vi "624 Detect Retroreflective Vision Totes.vi"(7 "Limit %":dbl=0.5 format="%#_13g", 8 "Filter Settings":T2, 9 "Ring Light Color":T4={"Hue"={101.37467765958063, 64.10933859299683}, "Sat"={88.03571428571429, 255.0}, "Val"={133.57142857142858, 255.0}} {"Hue" scale=0.0..255.0 scale format="%#_3g"}, 10 "Image Src":T3, 11 "Camera FOV width":dbl) -> (1 "Detected totes":T1[](array[typedef]), 2 "Masked":T3(plugin-control), 3 "Processed Img":T3(plugin-control))   [LabVIEW 2014]
uses:
  <vilib>/vision/Image Controls.llb/IMAQ Image.ctl
  Particle Filter Settings.ctl
  Vision Tote Data.ctl
  <vilib>/vision/NI_Vision_Development_Module.lvlib
panel:
  in  "Aspect Fudge Factor":dbl=1.0
  out "ms to process":u32
  out "Particles":i32
  # "Instructions:\nUse Source to select image files from a directory or use a USB or IP camera connected to your laptop.\nUse the Color of a ring light to threshold and build particles. Adjust calibration if needed.\nSmall modifications to the diagram will allow for intensity processing instead of color.\nAnnotations show the rectangle and the scores from top to bottom."
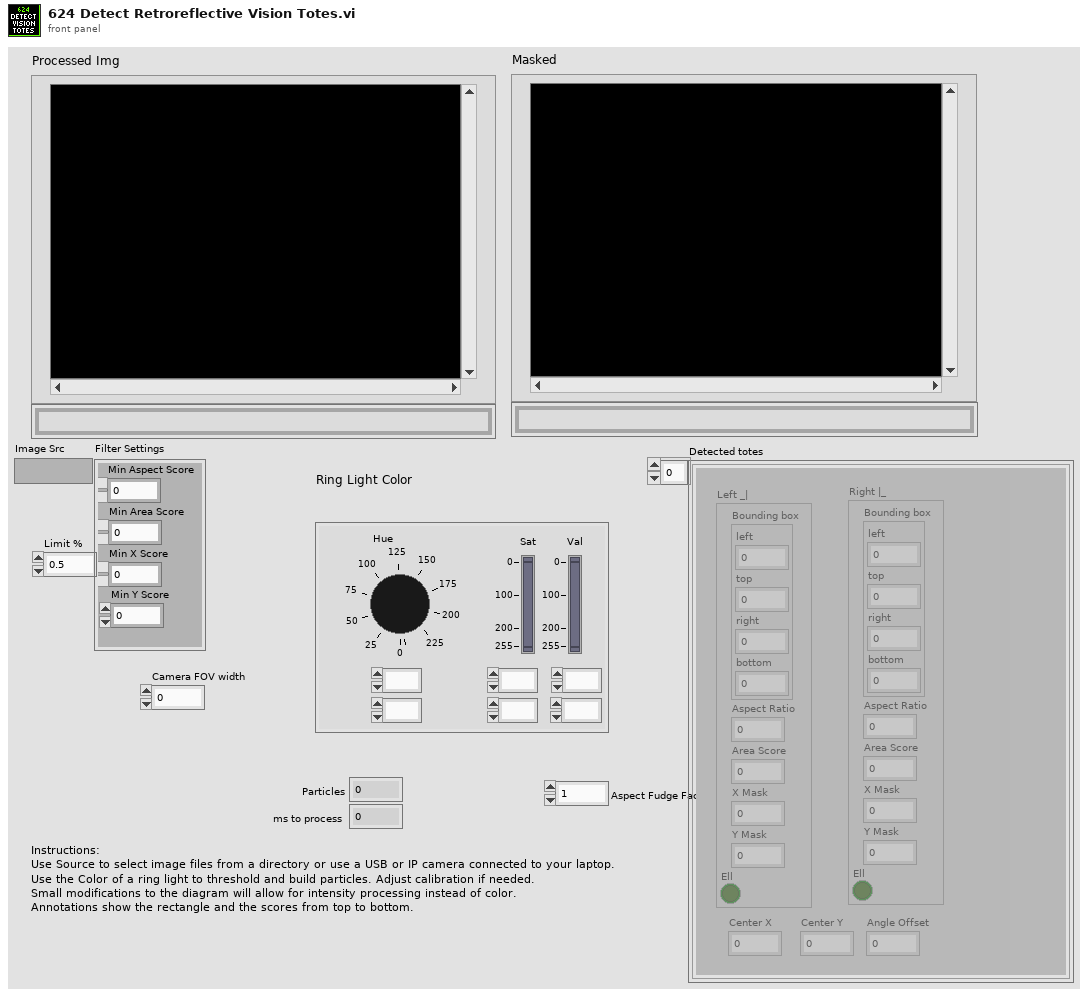
[diagram p1: front panel]
types:
  T1 = typedef "Vision Tote Data.ctl" = cluster{"Left _|":cluster{"Bounding box":cluster{"left":dbl, "top":dbl, "right":dbl, "bottom":dbl}, "Aspect Ratio":dbl, "Area Score":dbl, "X Mask":dbl, "Y Mask":dbl, "Ell":bool}, "Right |_":cluster{"Bounding box":cluster{"left":dbl, "top":dbl, "right":dbl, "bottom":dbl}, "Aspect Ratio":dbl, "Area Score":dbl, "X Mask":dbl, "Y Mask":dbl, "Ell":bool}, "Center X":dbl, "Center Y":dbl, "Angle Offset":dbl}
  T2 = typedef "Particle Filter Settings.ctl" = cluster{"Min Aspect Score":dbl, "Min Area Score":dbl, "Min X Score":dbl, "Min Y Score":dbl}
  T3 = typedef "IMAQ Image.ctl" = refnum<image>
  T4 = cluster{"Hue":cluster{dbl, dbl}, "Sat":cluster{dbl, dbl}, "Val":cluster{dbl, dbl}}
  T5 = typedef "Particle Parameters" = i32
  T6 = typedef "Image Type" = u32
  T7 = cluster{"Bounding box":cluster{"left":dbl, "top":dbl, "right":dbl, "bottom":dbl}, "Aspect Ratio":dbl, "Area Score":dbl, "X Mask":dbl, "Y Mask":dbl, "Ell":bool}[]
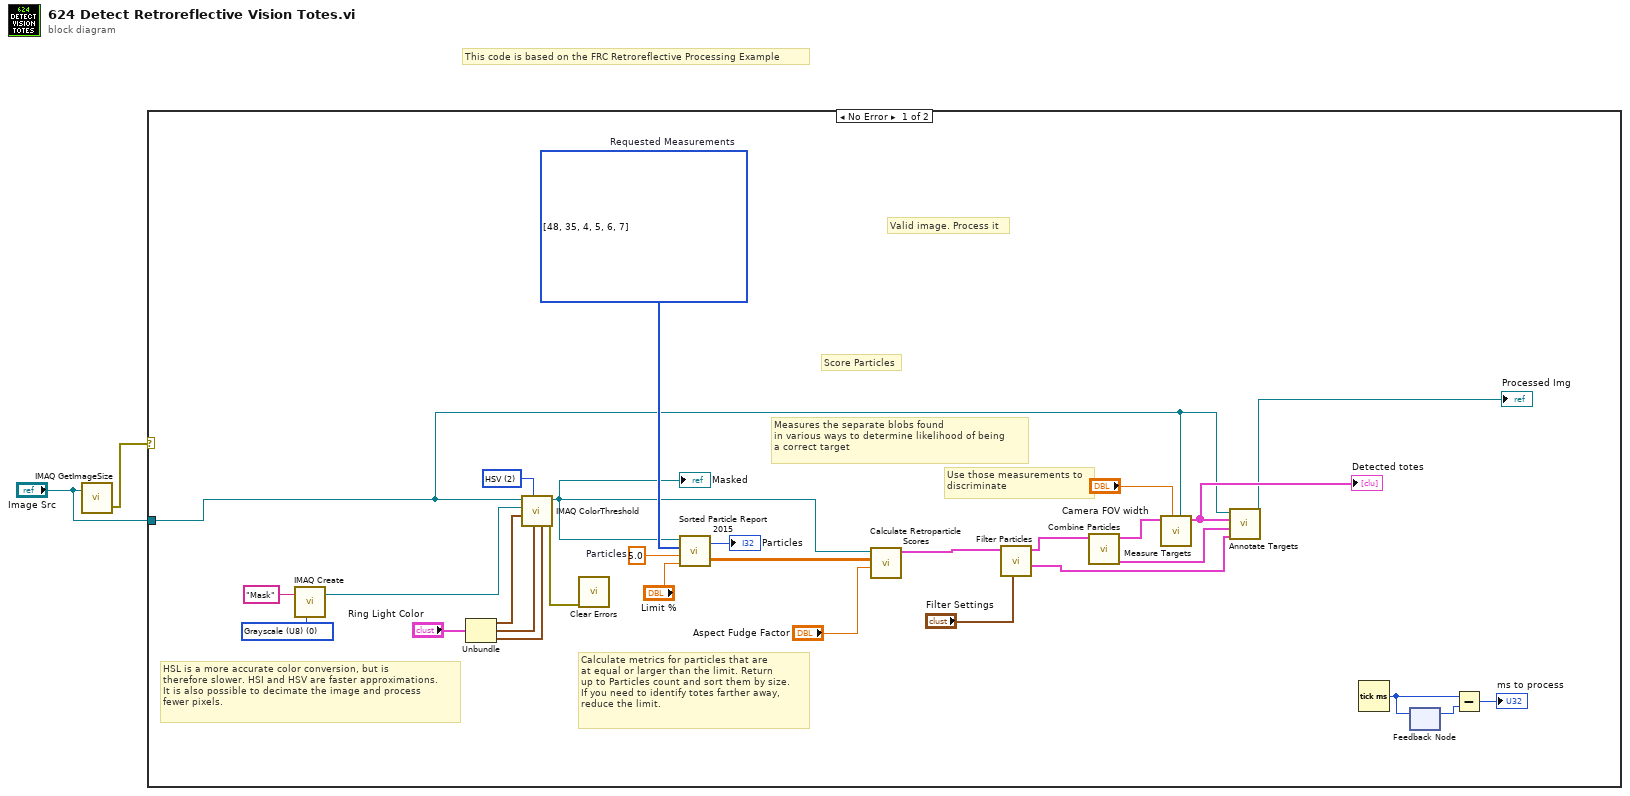
[diagram p0: block diagram]
diagram:
  # "This code is based on the FRC Retroreflective Processing Example"
  n1 = call "IMAQ GetImageSize"("Image"="Image Src") -> ("error out"=w1:errorcluster)  [unwired: 3 in, 2 out]
  n2 = case shown="No Error" w1 {
    tunnel: "Image Src" -> [w4 _]
    frame No Error {
      w22 = 5.0  # Particles
      w27 = u16 2 items=["RGB", "HSL", "HSV", "HSI"] ("Color Mode")
      w28 = T5[] [48, 35, 4, 5, 6, 7] items=["Center of Mass X", "Center of Mass Y", "First Pixel X", "First Pixel Y", "Bounding Rect Left", "Bounding Rect Top", "Bounding Rect Right", "Bounding Rect Bottom", "Max Feret Diameter Start X", "Max Feret Diameter Start Y", "Max Feret Diameter End X", "Max Feret Diameter End Y", "Max Horiz. Segment Length Left", "Max Horiz. Segment Length Right", "Max Horiz. Segment Length Row", "-", "Bounding Rect Width", "Bounding Rect Height", "Bounding Rect Diagonal", "Perimeter", "Convex Hull Perimeter", "Holes' Perimeter", "Max Feret Diameter", "Equivalent Ellipse Major Axis", "Equivalent Ellipse Minor Axis", "Equivalent Ellipse Minor Axis (Feret)", "Equivalent Rect Long Side", "Equivalent Rect Short Side", "Equivalent Rect Diagonal", "Equivalent Rect Short Side (Feret)", "Average Horiz. Segment Length", "Average Vert. Segment Length", "Hydraulic Radius", "Waddel Disk Diameter", "-", "Area", "Holes' Area", "Particle & Holes' Area", "Convex Hull Area", "Image Area", "-", "Number of Holes", "Number of Horiz. Segments", "Number of Vert. Segments", "-", "Orientation", "Max Feret Diameter Orientation", "-", "% Area/Image Area", "% Area/(Particle & Holes' Area)", "Ratio of Equivalent Ellipse Axes", "Ratio of Equivalent Rect Sides", "-", "Elongation Factor", "Compactness Factor", "Heywood Circularity Factor", "Type Factor", "-", "Sum X", "Sum Y", "Sum XX", "Sum XY", "Sum YY", "Sum XXX", "Sum XXY", "Sum XYY", "Sum YYY", "-", "Moment of Inertia XX", "Moment of Inertia XY", "Moment of Inertia YY", "Moment of Inertia XXX", "Moment of Inertia XXY", "Moment of Inertia XYY", "Moment of Inertia YYY", "Norm. Moment of Inertia XX", "Norm. Moment of Inertia XY", "Norm. Moment of Inertia YY", "Norm. Moment of Inertia XXX", "Norm. Moment of Inertia XXY", "Norm. Moment of Inertia XYY", "Norm. Moment of Inertia YYY", "Hu Moment 1", "Hu Moment 2", "Hu Moment 3", "Hu Moment 4", "Hu Moment 5", "Hu Moment 6", "Hu Moment 7"]  # Requested Measurements
      w31 = T6 0 items=["Grayscale (U8)", "Grayscale (I16)", "Grayscale (SGL)", "Complex (CSG)", "RGB (U32)", "HSL (U32)", "RGB (U64)", "Grayscale (U16)"] ("Image Type")
      # "Use those measurements to\ndiscriminate"
      # "Measures the separate blobs found\nin various ways to determine likelihood of being\na correct target"
      # "Calculate metrics for particles that are\nat equal or larger than the limit. Return\nup to Particles count and sort them by size.\nIf you need to identify totes farther away,\nreduce the limit."
      # "Score Particles"
      # "HSL is a more accurate color conversion, but is\ntherefore slower. HSI and HSV are faster approximations.\nIt is also possible to decimate the image and process\nfewer pixels."
      # "Valid image. Process it"
      n3 = call "IMAQ Create"("Image Name"="Mask", "Image Type"=w31) -> ("New Image"=w29:T3)  [unwired: 2 in, 2 out]
      n4 = Unbundle("Ring Light Color") -> ("Hue"=w26:cluster{dbl, dbl}, "Sat"=w25:cluster{dbl, dbl}, "Val"=w24:cluster{dbl, dbl})
      n5 = call "IMAQ ColorThreshold"("Blue or Luma or Val or Inten Range"=w24, "Green or Sat Range"=w25, "Color Mode"=w27, "Red or Hue Range"=w26, "Image Dst"=w29, "Image Src"=w4) -> ("error out"=w3:errorcluster, "Image Dst Out"=w10:T3)  [unwired: 4 in]
      "Masked" <- w10
      n6 = call <vilib>:"Clear Errors.vi"("error in (no error)"=w3) -> ()  [unwired: 5 in, 2 out]
      n7 = call "Sorted Particle Report 2015.vi"("Min Area Size %"="Limit %", "Particle Count Limit"=w22, "Pixel Measurements"=w28, "Image in"=w10) -> ("Sorted Data"=w14:dbl[][], "Particles"=→"Particles":i32)
      n8 = call "Calculate Retroparticle Scores.vi"("Aspect Fudge Factor"="Aspect Fudge Factor", "Sorted Data"=w14, "Image in"=w10) -> ("Scores"=w16:T7)  [unwired: 8 in]
      n9 = call "Filter Particles.vi"("Filter Settings"="Filter Settings", "Scores in"=w16) -> ("Rejected particles out"=w7:T7, "Good particles out"=w12:T7)  [unwired: 8 in]
      n10 = call "Combine Particles.vi"("Good particles in"=w12) -> ("Unpaired particles"=w8:T7, "Unmeasured Targets"=w11:T1[])  [unwired: 9 in]
      n11 = call "Measure Targets.vi"("Image"=w4, "FOV width"="Camera FOV width", "Unmeasured Targets in"=w11) -> ("Measured Targets out"=w9:T1[])  [unwired: 8 in]
      "Detected totes" <- w9
      n12 = call "Annotate Targets.vi"("Rejected particles"=w7, "Unpaired particles"=w8, "Measured Targets in"=w9, "Refnum in"=w4) -> ("Refnum out"=→"Processed Img":T3)  [unwired: 7 in]
      n13 = Tick Count (ms)() -> (millisecond timer value=w18:u32)
      n14 = feedback #1() -> (w19:u32)  [unwired: 1 in]
      n15 = feedback-in #1(w18) -> ()
      n16 = Subtract(x=w18, y=w19) -> (x-y=→"ms to process":u32)
    }
    frame Error {
      # "Invalid image. Don't bother processing"
    }
  }
